vi "Copy .LLB to NI VeriStand dir.vi"(5 "Files Generated by Build":path[](array[path]), 6 "Top Level/Always Included VIs":path[](array[path]), 7 "Destination Path":path, 8 "error in (no error)":errorcluster, 9 "Target Name":string, 10 "Build Specification Name":string, 11 "Project Path":path) -> (0 "error out":errorcluster)   [LabVIEW 2027]
doc: "This VI is called after each run of a build specification. The VI will copy the generated LLB (Engine or System Explorer) into the VeriStand Custom Device folder (...\\Documents\\National Instruments\\NI VeriStand 2013...)."
uses:
  <vilib>/Utility/sysdir.llb/System Directory Type.ctl
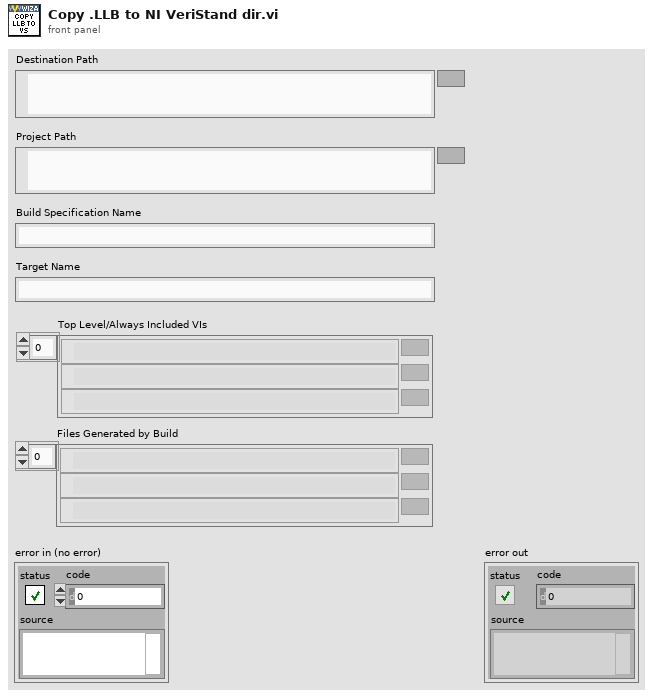
[diagram p1: front panel]
types:
  T1 = typedef "System Directory Type.ctl" = i32
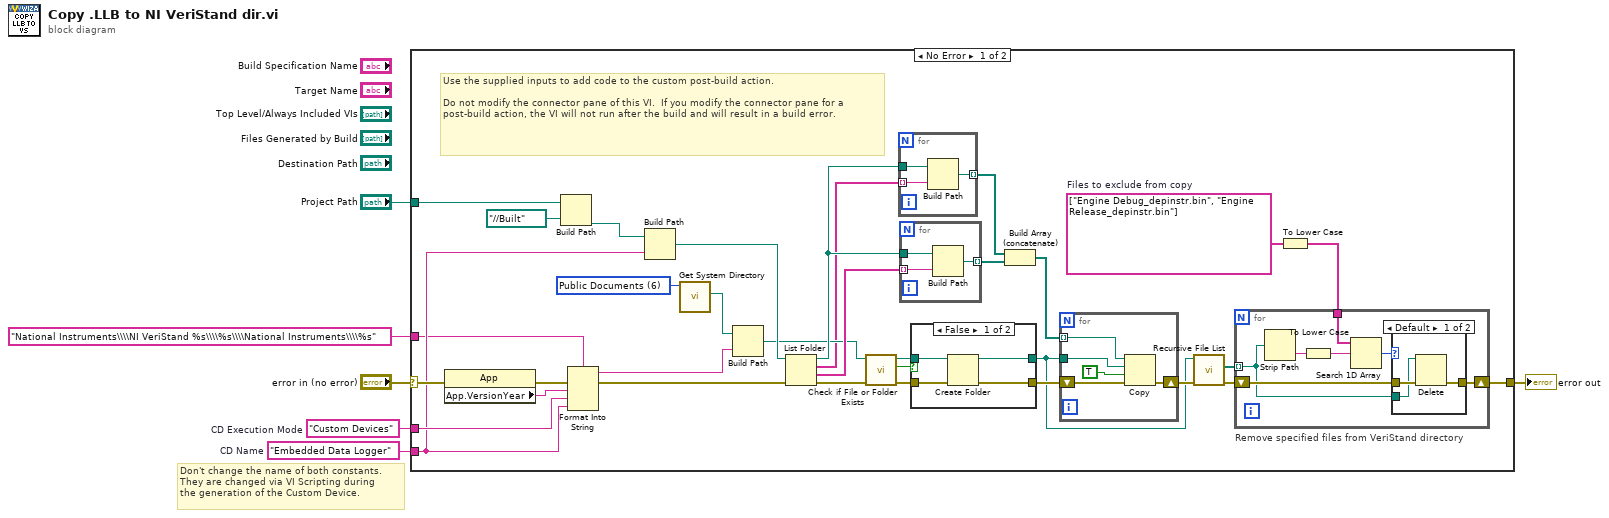
[diagram p0: block diagram]
diagram:
  w3 = "Embedded Data Logger"  # CD Name
  w4 = "Custom Devices"  # CD Execution Mode
  # "Don't change the name of both constants.\nThey are changed via VI Scripting during\nthe generation of the Custom Device."
  n1 = case shown="No Error" "error in (no error)" {
    selector: "error in (no error)" -> [w21 w68]
    tunnel: [w8 w68] -> w2
    tunnel: "Project Path" -> [w17 _]
    tunnel: w4 -> [w22 _]
    tunnel: w3 -> [w19 _]
    tunnel: "National Instruments\\\\NI VeriStand %s\\\\%s\\\\National Instruments\\\\%s" ("name or relative path") -> [w7 _]
    frame No Error {
      w14 = string[] ["Engine Debug_depinstr.bin", "Engine Release_depinstr.bin"]  # Files to exclude from copy
      w26 = T1 6 items=["User Home"=0, "User Desktop"=1, "User Documents"=2, "User Application Data"=3, "User Preferences"=4, "User Temporary"=5, "Public Documents"=6, "Public Application Data"=7, "Public Preferences"=8, "Public Cache"=13, "System Core Libraries"=9, "System Installed Libraries"=10, "Application Files"=11, "Boot Volume Root"=12] ("system directory type")
      # "Use the supplied inputs to add code to the custom post-build action.\n\nDo not modify the connector pane of this VI.  If you modify the connector pane for a post-build action, the VI will not run after the build and will result in a build error."
      n2 = property class="App"(error in=w21) -> (error out=w25:errorcluster, "App.VersionYear"=w24:string)  [unwired: 1 in, 1 out]
      n3 = Build Path(base path=w17, name or relative path=path "../../Built") -> (appended path=w29:path)
      n4 = Format Into String(format string=w7, error in=w25, w24, w22, w19) -> (resulting string=w28:string, error out=w20:errorcluster)  [unwired: 1 in]
      n5 = Build Path(base path=w29, name or relative path=w19) -> (appended path=w31:path)
      n6 = call <vilib>:"Get System Directory.vi"("system directory type"=w26) -> ("system directory"=w27:path)  [unwired: 10 in]
      n7 = Build Path(base path=w27, name or relative path=w28) -> (appended path=w23:path)
      n8 = List Folder(path=w31, error in=w20) -> (path out=w33:path, filenames=w15:string[], folder names=w34:string[], error out=w30:errorcluster)  [unwired: 2 in]
      n9 = call <vilib>:"Check if File or Folder Exists.vi"("error in (no error)"=w30, "path"=w23) -> ("error out"=w35:errorcluster, "file or folder exists?"=w37:bool, "dup path"=w36:path)  [unwired: 7 in]
      n10 = for {
        tunnel: w15 -> [w66] mode=indexing
        tunnel: w33 -> [w67]
        tunnel: [w65] -> w39 mode=indexing
        n11 = Build Path(base path=w67, name or relative path=w66) -> (appended path=w65:path)
      }
      n12 = for {
        tunnel: w34 -> [w63] mode=indexing
        tunnel: w33 -> [w64]
        tunnel: [w62] -> w32 mode=indexing
        n13 = Build Path(base path=w64, name or relative path=w63) -> (appended path=w62:path)
      }
      n14 = case shown="False" w37 {
        tunnel: w36 -> [w54 w56]
        tunnel: w35 -> [w53 w55]
        tunnel: [w52 w56] -> w9
        tunnel: [w51 w55] -> w16
        frame False {
          n15 = Create Folder(path (use dialog)=w54, error in=w53) -> (created path=w52:path, error out=w51:errorcluster)  [unwired: 1 in, 1 out]
        }
        frame True {
        }
      }
      n16 = Build Array (concatenate)(w39, w32) -> (w38:path[])
      n17 = for {
        tunnel: w38 -> [w58] mode=indexing
        shift-right: [w59] -> w10
        shift-left: w16 -> [w60]
        tunnel: w9 -> [w57]
        n18 = Copy(8:w60, 9:TRUE ("overwrite (F)"), 10:w57, 11:w58) -> (0:w59:errorcluster)  [unwired: 1 in, 2 out]
      }
      n19 = call <vilib>:"Recursive File List.vi"("error in (no error)"=w10, "Folder Path"=w9) -> ("error out"=w13:errorcluster, "All Files in Dir"=w12:path[])  [unwired: 5 in, 3 out]
      n20 = To Lower Case(string=w14) -> (all lower case string=w11:string[])
      n21 = for "Remove specified files from VeriStand directory" {
        shift-right: [w41] -> w8
        shift-left: w13 -> [w43]
        tunnel: w12 -> [w40] mode=indexing
        tunnel: w11 -> [w44]
        n22 = Strip Path(path=w40) -> (name=w46:string)  [unwired: 1 out]
        n23 = To Lower Case(string=w46) -> (all lower case string=w45:string)
        n24 = Search 1D Array(1D array=w44, element=w45) -> (index of element=w42:i32)  [unwired: 1 in]
        n25 = case shown="Default" w42 {
          tunnel: w43 -> [w49 w50]
          tunnel: [w48 w50] -> w41
          tunnel: w40 -> [w47 _]
          frame Default {
            n26 = Delete(path (use dialog)=w47, error in=w49) -> (error out=w48:errorcluster)  [unwired: 3 in, 2 out]
          }
          frame -1 {
          }
        }
      }
    }
    frame Error {
    }
  }
  "error out" <- w2
